vi "FdxCmdRxGlobalStatisticsCvi.vi"(8 "error in":errorcluster, 9 "Control":u32(ring) items=["FDX_RX_GS_RES_NO_CNT", "FDX_RX_GS_RES_ALL_CNT", "FDX_RX_GS_RES_ERR_CNT"], 11 "InstrumentHandle_port":u32) -> (0 "error out":errorcluster, 1 "GlobalStat Out":T1, 3 "InstrumentHandle_port":u32)   [LabVIEW 2020, in "AIM664LV.lvlib"]
doc: "Get the busload measurement values to give an indicator about the full bus traffic over all Virtual Links."
uses:
  AIM664LV.lvlib
  AFDX_LibraryAdmin/FdxGlobalDllPath.vi
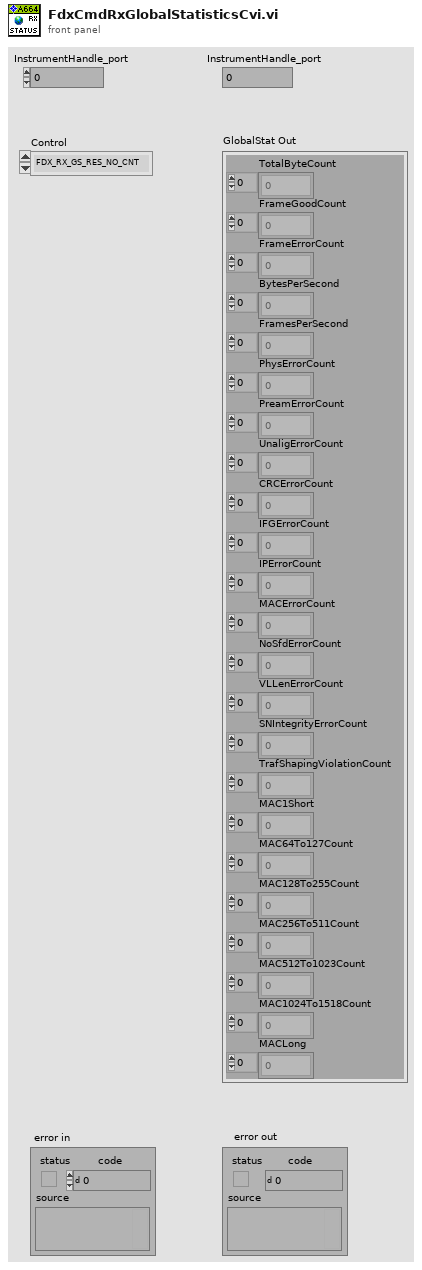
[diagram p1: front panel]
types:
  T1 = cluster{"TotalByteCount":u32[], "FrameGoodCount":u32[], "FrameErrorCount":u32[], "BytesPerSecond":u32[], "FramesPerSecond":u32[], "PhysErrorCount":u32[], "PreamErrorCount":u32[], "UnaligErrorCount":u32[], "CRCErrorCount":u32[], "IFGErrorCount":u32[], "IPErrorCount":u32[], "MACErrorCount":u32[], "NoSfdErrorCount":u32[], "VLLenErrorCount":u32[], "SNIntegrityErrorCount":u32[], "TrafShapingViolationCount":u32[], "MAC1Short":u32[], "MAC64To127Count":u32[], "MAC128To255Count":u32[], "MAC256To511Count":u32[], "MAC512To1023Count":u32[], "MAC1024To1518Count":u32[], "MACLong":u32[]}
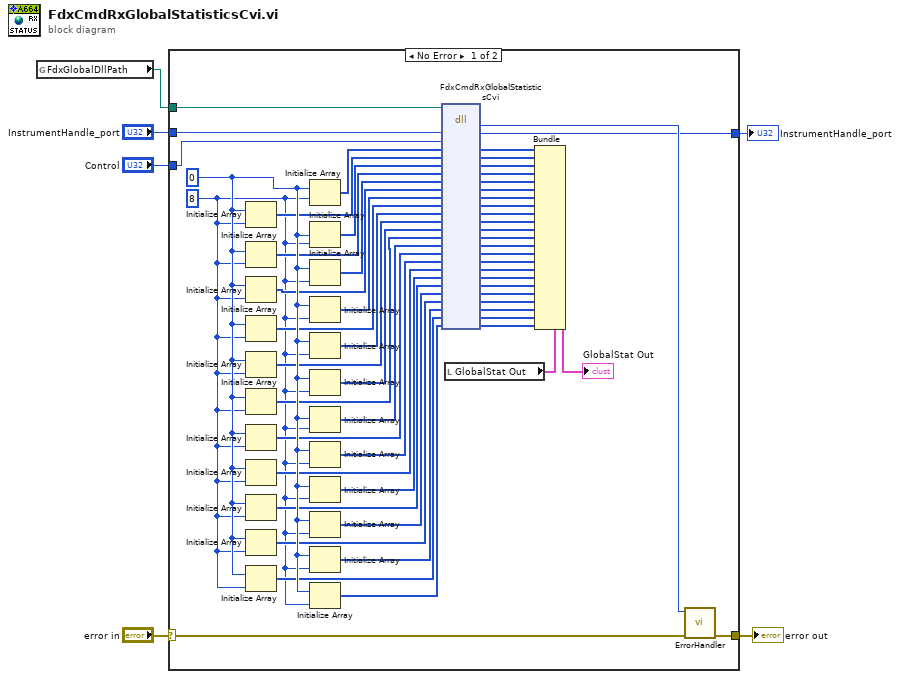
[diagram p0: block diagram]
diagram:
  n1 = global read "FdxGlobalDllPath.vi" "FdxGlobalDllPath"() -> (w4:path)
  n2 = case shown="No Error" "error in" {
    selector: "error in" -> [w62 w65]
    tunnel: [w63 w65] -> w6
    tunnel: w4 -> [w10 _]
    tunnel: [w9 w64] -> w3
    tunnel: "InstrumentHandle_port" -> [w8 w64]
    tunnel: "Control" -> [w7 _]
    frame No Error {
      w48 = u32 0 ("element")
      w24 = 8 ("dimension size")
      n3 = Initialize Array(w48, w24) -> (w46:u32[])
      n4 = Initialize Array(w48, w24) -> (w44:u32[])
      n5 = Initialize Array(w48, w24) -> (w43:u32[])
      n6 = Initialize Array(w48, w24) -> (w40:u32[])
      n7 = Initialize Array(w48, w24) -> (w38:u32[])
      n8 = Initialize Array(w48, w24) -> (w36:u32[])
      n9 = Initialize Array(w48, w24) -> (w34:u32[])
      n10 = Initialize Array(w48, w24) -> (w32:u32[])
      n11 = Initialize Array(w48, w24) -> (w30:u32[])
      n12 = Initialize Array(w48, w24) -> (w28:u32[])
      n13 = Initialize Array(w48, w24) -> (w26:u32[])
      n14 = Initialize Array(w48, w24) -> (w47:u32[])
      n15 = Initialize Array(w48, w24) -> (w45:u32[])
      n16 = Initialize Array(w48, w24) -> (w42:u32[])
      n17 = Initialize Array(w48, w24) -> (w41:u32[])
      n18 = Initialize Array(w48, w24) -> (w39:u32[])
      n19 = Initialize Array(w48, w24) -> (w37:u32[])
      n20 = Initialize Array(w48, w24) -> (w35:u32[])
      n21 = Initialize Array(w48, w24) -> (w33:u32[])
      n22 = Initialize Array(w48, w24) -> (w31:u32[])
      n23 = Initialize Array(w48, w24) -> (w29:u32[])
      n24 = Initialize Array(w48, w24) -> (w27:u32[])
      n25 = Initialize Array(w48, w24) -> (w25:u32[])
      n26 = dll-call lib="aim_fdx.19.dll" fn="FdxCmdRxGlobalStatisticsCvi"(path in=w10, "InstrumentHandle"=w8, "Control"=w7, "TotalByteCount"=w47, "FrameGoodCount"=w46, "FrameErrorCount"=w45, "BytesPerSecond"=w44, "FramesPerSecond"=w42, "PhysErrorCount"=w43, "PreamErrorCount"=w41, "UnaligErrorCount"=w40, "CRCErrorCount"=w39, "IFGErrorCount"=w38, "IPErrorCount"=w37, "MACErrorCount"=w36, "NoSfdErrorCount"=w35, "VLLenErrorCount"=w34, "SNIntegrityErrorCount"=w33, "TrafShapingViolationCount"=w32, "MAC1Short"=w31, "MAC64To127Count"=w30, "MAC128To255Count"=w29, "MAC256To511Count"=w28, "MAC512To1023Count"=w27, "MAC1024To1518Count"=w26, "MACLong"=w25) -> ("status"=w61:i32, "InstrumentHandle"=w9:u32, "TotalByteCount"=w60:u32[], "FrameGoodCount"=w59:u32[], "FrameErrorCount"=w58:u32[], "BytesPerSecond"=w57:u32[], "FramesPerSecond"=w56:u32[], "PhysErrorCount"=w55:u32[], "PreamErrorCount"=w54:u32[], "UnaligErrorCount"=w53:u32[], "CRCErrorCount"=w52:u32[], "IFGErrorCount"=w50:u32[], "IPErrorCount"=w49:u32[], "MACErrorCount"=w23:u32[], "NoSfdErrorCount"=w22:u32[], "VLLenErrorCount"=w21:u32[], "SNIntegrityErrorCount"=w20:u32[], "TrafShapingViolationCount"=w19:u32[], "MAC1Short"=w18:u32[], "MAC64To127Count"=w17:u32[], "MAC128To255Count"=w16:u32[], "MAC256To511Count"=w15:u32[], "MAC512To1023Count"=w14:u32[], "MAC1024To1518Count"=w13:u32[], "MACLong"=w12:u32[])  [unwired: 3 in, 2 out]
      n27 = local read "GlobalStat Out"() -> (w11:T1)
      n28 = Bundle(cluster=w11, "TotalByteCount"=w60, "FrameGoodCount"=w59, "FrameErrorCount"=w58, "BytesPerSecond"=w57, "FramesPerSecond"=w56, "PhysErrorCount"=w55, "PreamErrorCount"=w54, "UnaligErrorCount"=w53, "CRCErrorCount"=w52, "IFGErrorCount"=w50, "IPErrorCount"=w49, "MACErrorCount"=w23, "NoSfdErrorCount"=w22, "VLLenErrorCount"=w21, "SNIntegrityErrorCount"=w20, "TrafShapingViolationCount"=w19, "MAC1Short"=w18, "MAC64To127Count"=w17, "MAC128To255Count"=w16, "MAC256To511Count"=w15, "MAC512To1023Count"=w14, "MAC1024To1518Count"=w13, "MACLong"=w12) -> (→"GlobalStat Out":T1)
      n29 = call "ErrorHandler.vi"("error in"=w62, "AIM Error"=w61) -> ("error out"=w63:errorcluster)  [unwired: 9 in]
    }
    frame Error {
    }
  }
  "error out" <- w6
  "InstrumentHandle_port" <- w3
